vi "VMSemaphoreRelease.vi"(8 "error in (no error)":errorcluster, 10 "VariableManager":refnum<class "VariableManager.lvclass">, 11 "VariableManagerRef in":refnum<vi>) -> (0 "error out":errorcluster, 3 "VariableManagerRef out":refnum<vi>)   [LabVIEW 2013, in "VariableManagerAPI.lvlib"]
doc: "VMSemaphoreAcquire.vi and VMSemaphoreRelease.vi ensure synchronous data operations on a reference to a VariableManager object.\n\nVMSemaphoreRelease.vi writes the given VariableManager object to the reference and release the object for next process that call VMSemaphoreAcquire.vi."
uses:
  VariableManagerAPI.lvlib
  VariableManager/VariableManager.lvclass
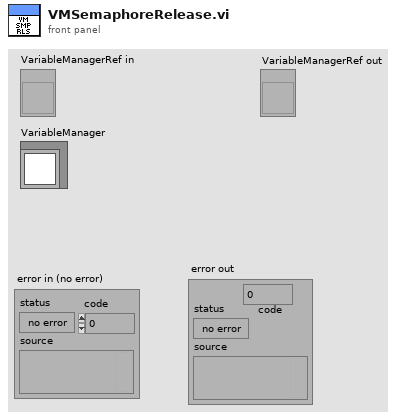
[diagram p1: front panel]
types:
  T1 = typedef "Semaphore RefNum" = refnum<k1>
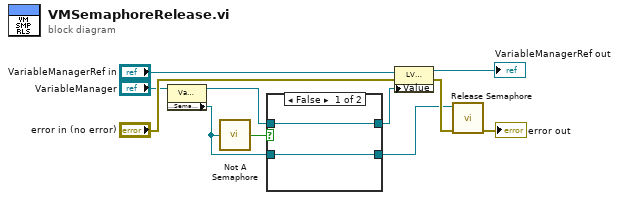
[diagram p0: block diagram]
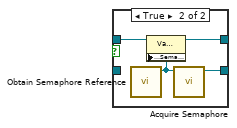
[diagram p2: hidden frame]
diagram:
  n1 = property class="VariableManager.lvclass"(reference="VariableManager") -> (reference out=w4:refnum<class "VariableManager.lvclass">, "Accessors:Semaphore"=w3:T1)  [unwired: 1 in, 1 out]
  n2 = call <vilib>:"Not A Semaphore.vi"("semaphore"=w3) -> ("not a semaphore"=w5:bool)
  n3 = case shown="False" w5 {
    tunnel: w4 -> [w13 w17]
    tunnel: [w13 w16] -> w2
    tunnel: w3 -> [w12 _]
    tunnel: [w12 w14] -> w1
    frame False {
    }
    frame True {
      n4 = call <vilib>:"Obtain Semaphore Reference.vi"() -> ("semaphore"=w15:T1)  [unwired: 5 in, 2 out]
      n5 = property class="VariableManager.lvclass"(reference=w17, "Accessors:Semaphore"=w15) -> (reference out=w16:refnum<class "VariableManager.lvclass">)  [unwired: 1 in, 1 out]
      n6 = call <vilib>:"Acquire Semaphore.vi"("semaphore"=w15) -> ("semaphore out"=w14:T1)  [unwired: 4 in, 2 out]
    }
  }
  n7 = property class="LVClassControl (strict)"(reference="VariableManagerRef in", error in="error in (no error)", "Value"=w2) -> (reference out=→"VariableManagerRef out":refnum<vi>, error out=w11:errorcluster)
  n8 = call <vilib>:"Release Semaphore.vi"("error in (no error)"=w11, "semaphore"=w1) -> ("error out"=→"error out":errorcluster)  [unwired: 4 in, 1 out]
